vi "reg_visu.vi"(7 "name":string="GM10", 9 "stop":bool, 10 "connect (T)":bool=TRUE) -> (0 "error out":errorcluster, 5 "This VI":refnum<vi>)   [LabVIEW 2019]
uses:
  Heating/ctl/Z_ind_heating.ctl
  Heating/ctl/Z_Hswitch/Z_Hswitch.xctl
  ctl/Y/Y.xctl
  Heating/ctl/Z_State.ctl
  Heating/ctl/Y_state.ctl
  Heating/ctl/ZM_State.ctl
  Heating/ctl/Y_source.ctl
  ctl/control param simple.ctl
  ctl/Y_state.ctl
  ctl/Y_short.ctl
  Inputs/Ctl/Parameter State short.ctl
  ctl/ZY_control_short.ctl
  ctl/Z_State.ctl
  45230f51-ed9d-4592-a49a-e0edfe92ddd1.vi
  fbc51cc2-a17d-4d51-90ca-ef1d5e9adb43.vi
  81bac83f-5a8a-4521-9bb9-45d0222ee4c6.vi
  Y_switch_control.vi
  Y Limiter_ext.vi
  Counter/Generator simplified.vi
  <vilib>/NI/AMC/Create Single Message.vi
  <vilib>/NI/AMC/Update Message Routing Info.vi
  <vilib>/NI/AMC/Read Termination Message.vi
  PID Output Rate Limiter Ext.vi
  PID Timing Estimation Ext.vi
  Heating/Global stop.vi
  <vilib>/NI/AMC/Send Message.vi
  <vilib>/NI/AMC/Globals.vi
  Heating/Heating.lvlib
  <vilib>/NI/AMC/AMC.lvlib
  control.lvlib
  Inputs/Inputs.lvlib
panel:
  out "PV 2":dbl(slide) scale=0.0..1.0
  in  "Button":bool
  in  "Y":dbl step=0.01 format="%.2f"
  in  "Scale max":dbl=1.0 format="%#_13g"
  in  "name 4":string="Осн."
  in  "Unit":enum16{"l/h", "m3/h"}(ring)
  in  "name 3":string="Осн."
  in  "t":dbl=10.5 caption="сек."
  in  "alarm val":dbl=3.01 caption="m3/h"
  in  "auto":dbl=15.888 caption="Зависимый"
  in  "k":dbl=1.459 caption="Коэфф"
  in  "Y_SP":cluster{dbl, dbl, dbl}(xcontrol)
  in  "message name":string="AI redefine"
  out "status":string
  in  "process":bool
  in  "state variables":cluster{"CurrentFile":path}
  out "JSON string":string
  in  "JSON":string
  in  "Write controls":bool
  out "T stage":dbl format="%<%M:%S>t"
  in  "ALRL1_reset":bool
  in  "ALRL2_reset":bool
  out "Z3 ind":T1
  in  "Z_Hswitch":bool(xcontrol)
  out "Z5 State":string
  # "Время установки"
  # "Аварийный"
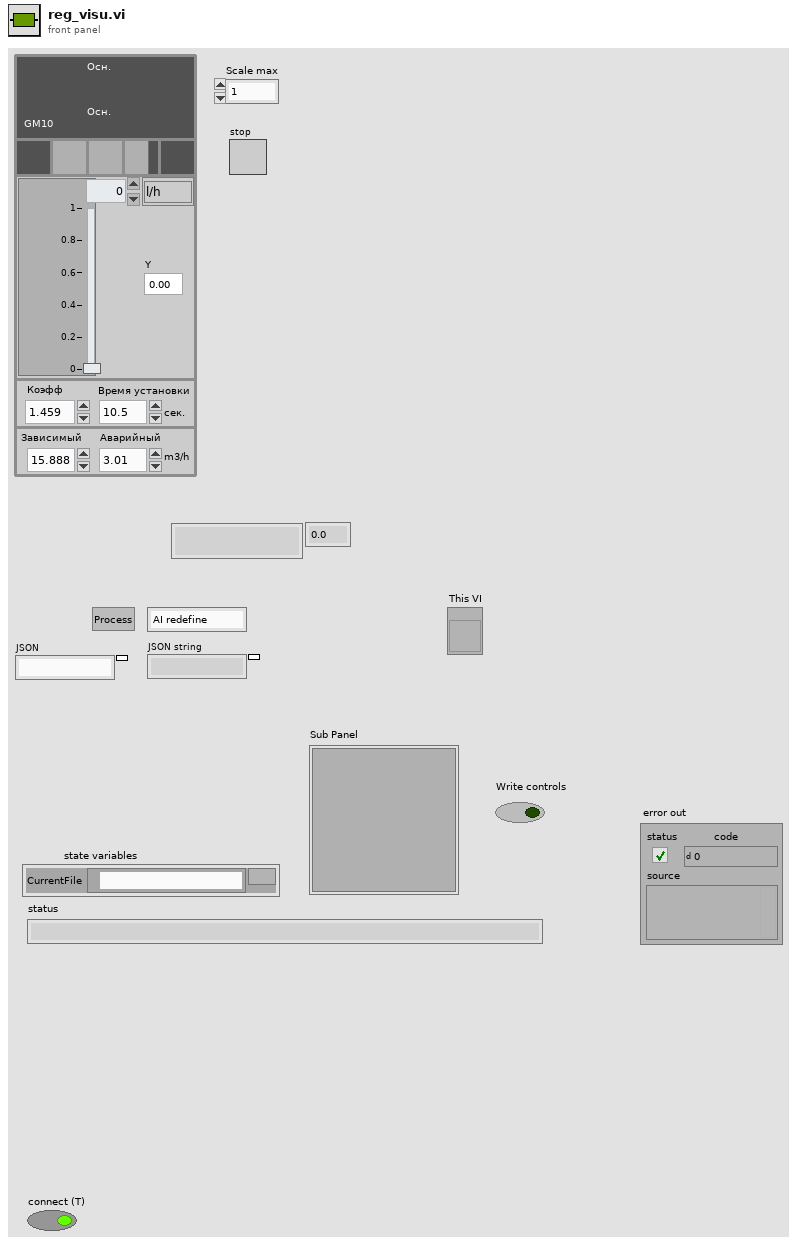
[diagram p1: front panel]
types:
  T1 = typedef "Heating.lvlib/Z_ind_heating.ctl" = u16
  T2 = typedef "AMC.lvlib/Message Queue.ctl" = refnum<queue>
  T3 = typedef "control.lvlib/ZY_control_short.ctl" = cluster{"Start":bool, "Z_HSw":u32, "Z_HSetState":T4, "Y_HSw":u32, "Y_HSetState":T5, "SP":dbl, "Y_H":dbl, "Y_A":dbl, "Reset_ALR":bool}
  T4 = typedef "control.lvlib/Z_State.ctl" = enum8{"initialization", "alarm", "disabled", "not ready", "stop ready", "reserv", "switched off", "reserv2", "switched on", "check", "on min", "decrease out", "on", "increase out", "on max"}
  T5 = typedef "control.lvlib/Y_state.ctl" = enum8{"initialize", "alarm", "min", "stop", "hand", "auto", "max"}
  T6 = typedef "control.lvlib/Y_short.ctl" = cluster{"Y_Source":u8, "Y_SetState":u8, "SP_Set":dbl, "SP":dbl, "PV":dbl, "PV_State":T7, "Y_preSet":dbl, "Y_Set":dbl, "Y":dbl, "Y_State":T7, "YB":bool}
  T7 = typedef "Inputs.lvlib/Parameter State short.ctl" = cluster{"code":i32, "visible":bool, "color":u32}
  T8 = cluster{"Y_HSw":u32, "Y_HSetState":T5, "Y_ASetState":T5, "Y_DSetState":T5}
  T9 = typedef "control.lvlib/control param simple.ctl" = cluster{"output high":dbl, "alr value":dbl, "output low":dbl, "output time (t)":dbl}
  T10 = typedef "Heating.lvlib/Y_source.ctl" = enum8{"initialize", "local disabled", "local hand", "hand", "auto", "dist"}
  T11 = cluster{"connect":bool, "SP_Source":T10, "SP_Set":dbl, "SP":dbl}
  T12 = typedef "Heating.lvlib/Y_state.ctl" = enum8{"initialize", "alarm", "min", "stop", "hand", "auto", "max"}
  T13 = typedef "Heating.lvlib/Z_State.ctl" = enum8{"initialization", "alarm", "disabled", "not ready", "stop ready", "reserv", "switched off", "reserv2", "switched on", "check", "on min", "decrease out", "on", "increase out", "on max"}
  T14 = typedef "Heating.lvlib/ZM_State.ctl" = enum8{"initialization", "stop", "start_cmd", "contactor_on_cmd", "heating", "on", "stop_cmd", "power_down", "contactor_off_cmd", "cooling", "restart_delay"}
  T15 = enum32{"Invalid Status", "Unconnected", "Active", "Idle", "Error", "Connecting"}
  T16 = typedef "LVDataSocketStatusTypeDef.ctl" = cluster{"Code":enum32{"Invalid Status", "Unconnected", "Active", "Idle", "Error", "Connecting"}, "Text":string}
  T17 = typedef "Y_Lim_ext_defs.ctl" = cluster{"reinitialize":bool, "SpLim_State":T18, "output":dbl, "Tick":u32, "output rate":dbl, "Y_Set":dbl, "Y_preSet":dbl}
  T18 = typedef "Y_Lim_State.ctl" = enum8{"initialization", "alarm", "stop", "decrease", "increase"}
  T19 = typedef "control.lvlib/Y.ctl" = cluster{"Y_Source":T20, "Y_SetState":T5, "SP_Set":dbl, "SP":dbl, "PV":dbl, "PV_State":T7, "Y_preSet":dbl, "Y_Set":dbl, "Y":dbl, "Y_State":T7, "YB":bool}
  T20 = typedef "control.lvlib/Y_source.ctl" = enum8{"initialize", "local disabled", "local hand", "hand", "auto", "dist"}
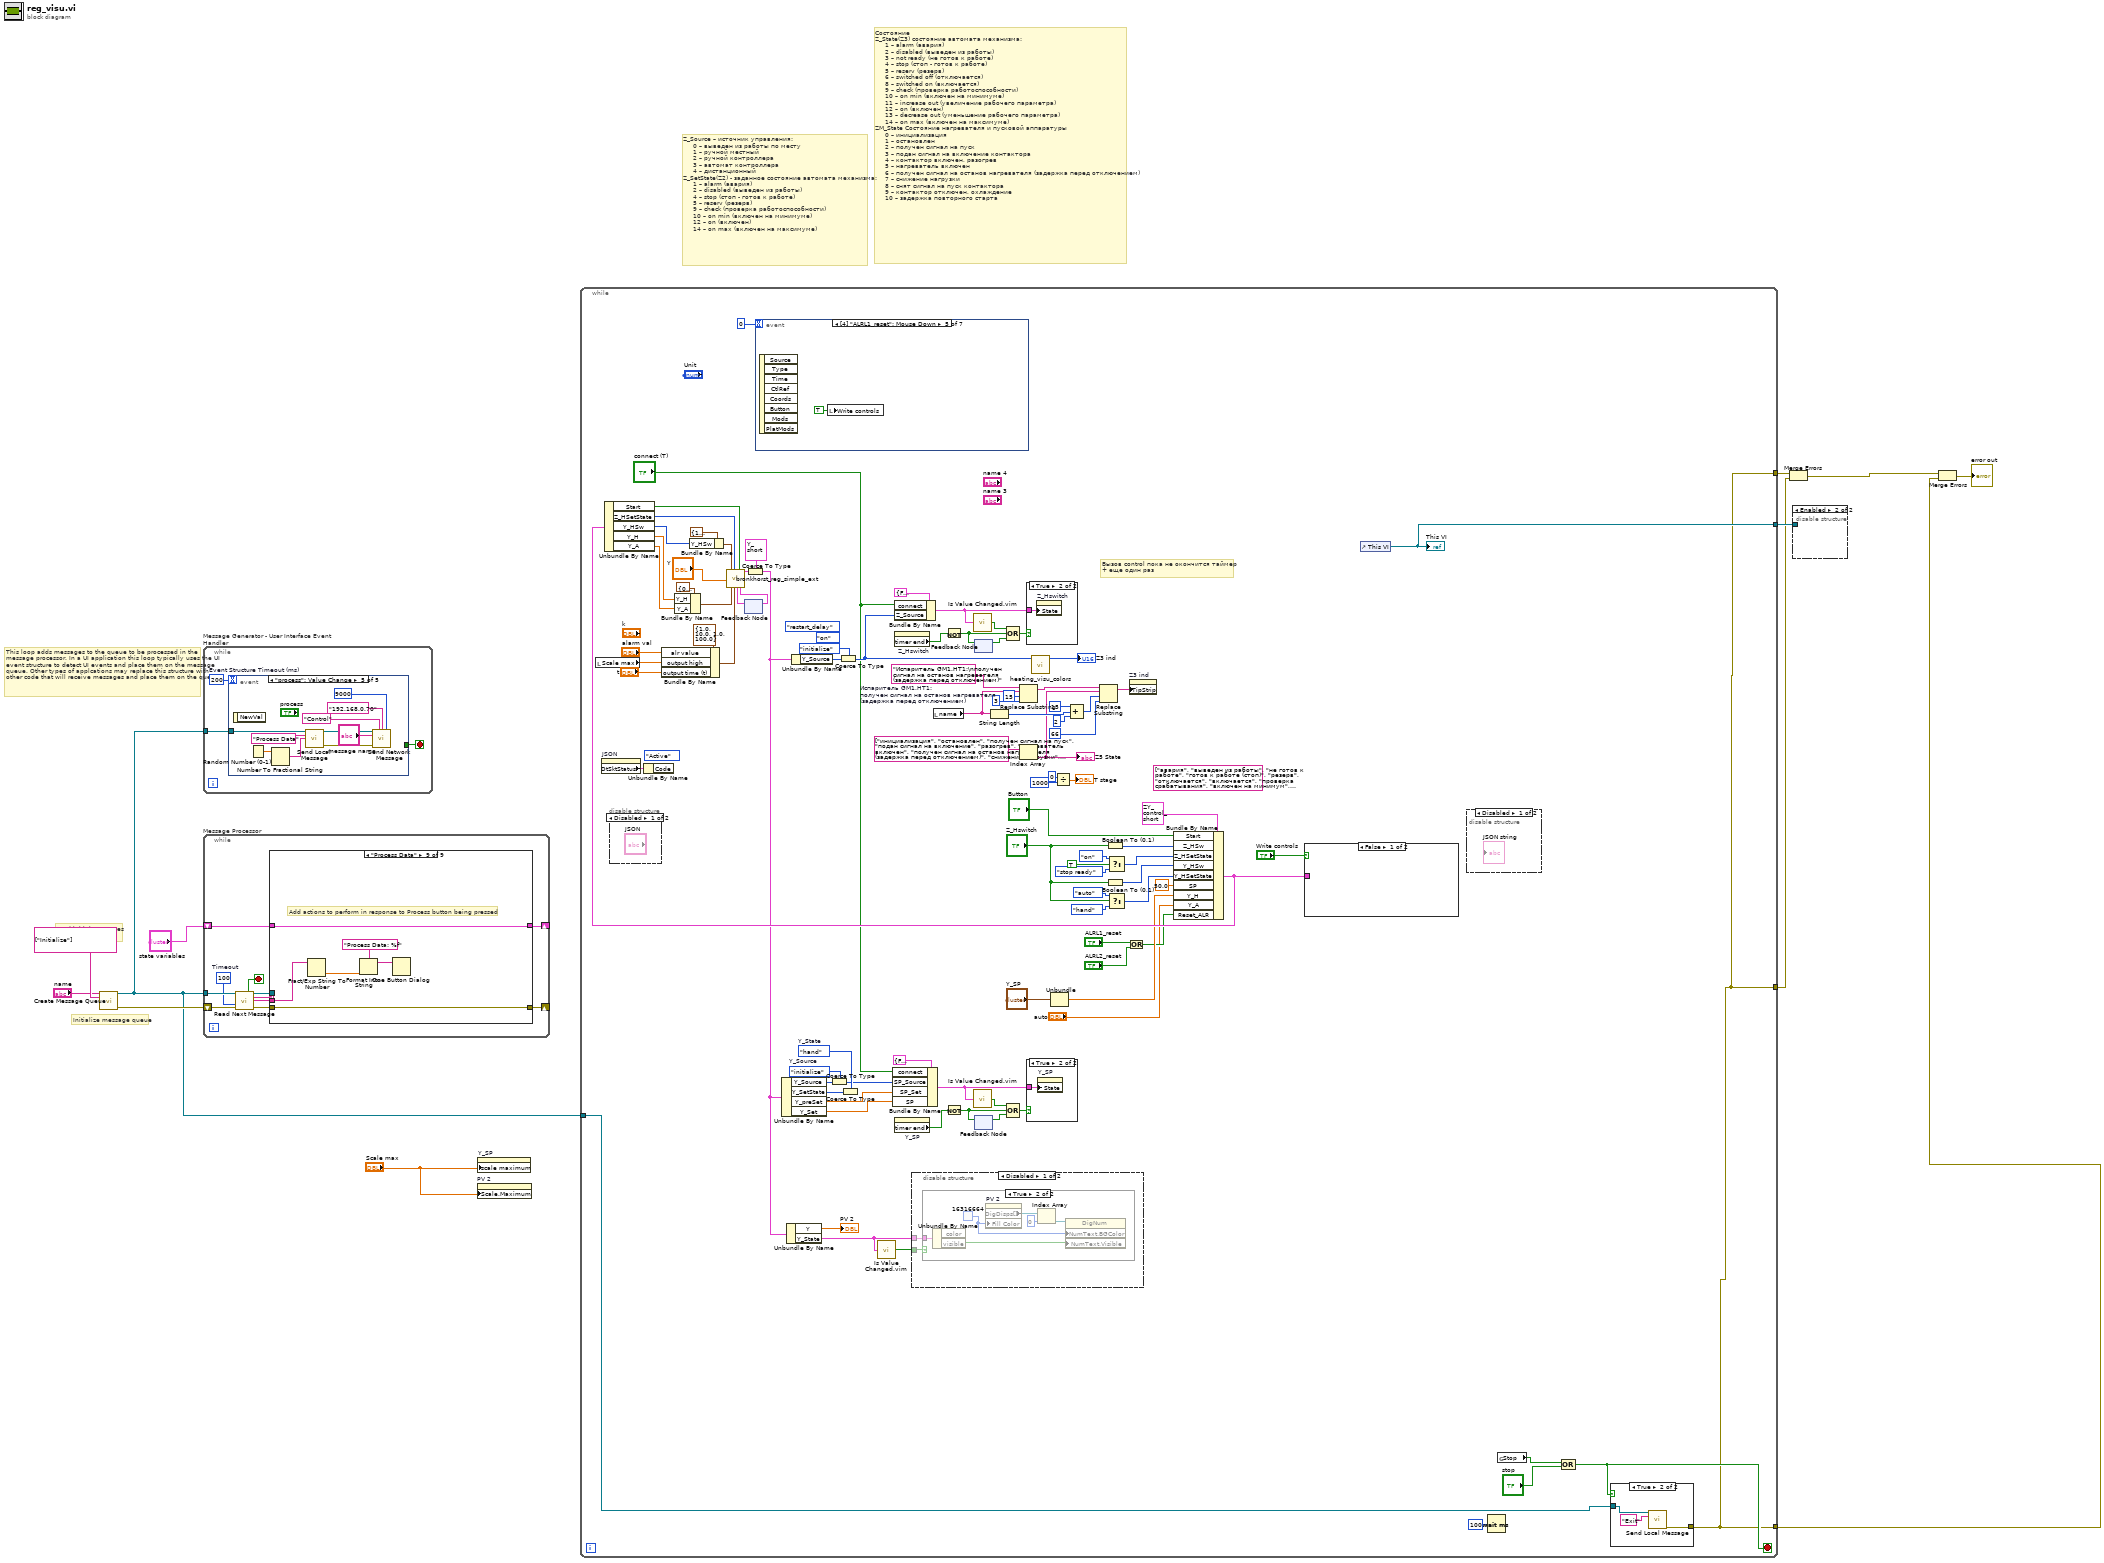
[diagram p0: block diagram]
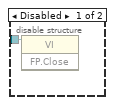
[diagram p2: hidden frame]
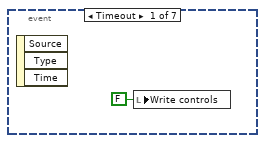
[diagram p8: hidden frame]
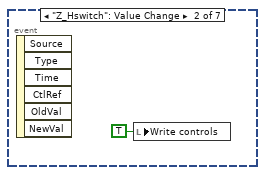
[diagram p9: hidden frame]
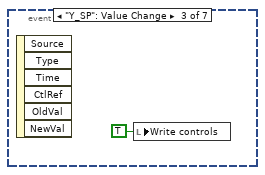
[diagram p10: hidden frame]
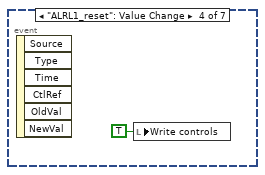
[diagram p11: hidden frame]
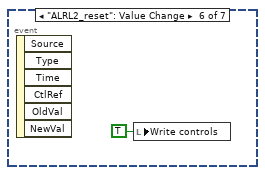
[diagram p12: hidden frame]
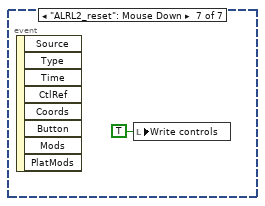
[diagram p13: hidden frame]
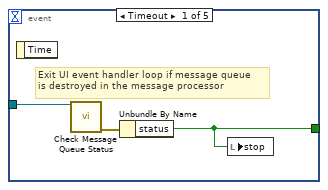
[diagram p17: hidden frame]
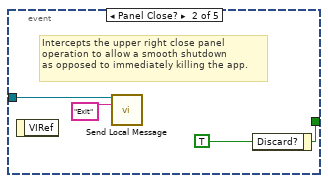
[diagram p18: hidden frame]
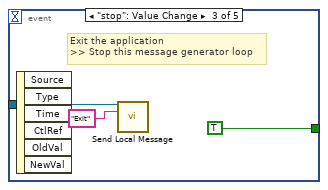
[diagram p19: hidden frame]
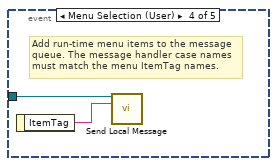
[diagram p20: hidden frame]
diagram:
  # "This loop adds messages to the queue to be processed in the message processor. In a UI application this loop typically uses the UI event structure to detect UI events and place them on the message queue. Other types of applcations may replace this structure with other code that will receive messages and place them on the queue."
  # "Initialize message queue"
  # "Load initial messages\non the queue"
  # "Состояние\nZ_State(Z3) состояние автомата механизма:\n     1 – alarm (авария)\n     2 – disabled (выведен из работы)\n     3 – not ready (не готов к работе)\n     4 – stop (стоп - готов к работе)\n     5 – reserv (резерв)\n     6 – switched off (отключается)\n     8 – switched on (включается)\n     9 – check (проверка работоспособности)\n     10 – on min (включен на минимуме)\n     11 – increase out (увеличение рабочего параметра)\n     12 – on (включен)\n     13 – decrease out (уменьшение рабочего параметра)\n     14 – on max (включен на максимуме)\nZM_State Состояние нагревателя и пусковой аппаратуры\n     0 – инициализация\n     1 – остановлен\n     2 – получен сигнал на пуск\n     3 – подан сигнал на включение контактора\n     4 – контактор включен, разогрев\n     5 – нагреватель включен\n     6 – получен сигнал на останов нагревателя (задержка перед отключением)\n     7 – снижение нагрузки\n     8 – снят сигнал на пуск контактора\n     9 – контактор отключен, охлаждение\n     10 – задержка повторного старта"
  # "Z_Source – источник управления:\n     0 – выведен из работы по месту\n     1 – ручной местный\n     2 – ручной контроллера\n     3 – автомат контроллера\n     4 – дистанционный\nZ_SetState(Z2) - заданное состояние автомата механизма:\n     1 – alarm (авария)\n     2 – disabled (выведен из работы)\n     4 – stop (стоп - готов к работе)\n     5 – reserv (резерв)\n     9 – check (проверка работоспособности)\n     10 – on min (включен на минимуме)\n     12 – on (включен)\n     14 – on max (включен на максимуме)"
  n1 = call <vilib>:"Create Message Queue.vi"("message queue name"="name", "initial message names"=string[] ["Initialize"]) -> ("message queue out"=w6:T2, "error out"=w8:errorcluster)  [unwired: 12 in]
  n2 = while "Message Generator - User Interface Event Handler" {
    tunnel: w6 -> [w13]
    stop <- w14 stop-if-true
    w15 = 200  # Event Structure Timeout (ms)
    n3 = event shown="[4] \"process\": Value Change" {
      selector: _ -> [_ _ _ _ _]
      dyn-events: _ -> [_ _ _ _ _]
      timeout: w15 -> [_ _ _ _ _]
      tunnel: [w16 w21 TRUE ("Discard?") _ _] -> w14
      tunnel: w13 -> [w17 w19 w22 w25 w36]
      event Timeout {
        # "Exit UI event handler loop if message queue\nis destroyed in the message processor"
        n4 = event-data() -> ()  [unwired: 2 out]
        n5 = call <vilib>:"Check Message Queue Status.vi"("message queue in"=w17) -> ("error out"=w18:errorcluster)  [unwired: 10 in, 4 out]
        n6 = Unbundle By Name(w18) -> ("status"=w16:bool)
        n7 = local write "stop"(w16) -> ()
      }
      event Panel Close? {
        w21 = TRUE ("Discard?")
        # "Intercepts the upper right close panel\noperation to allow a smooth shutdown\nas opposed to immediately killing the app."
        n8 = event-data() -> ()  [unwired: 2 out]
        n9 = call <vilib>:"Send Local Message.vi"("message queue in"=w19, "message name"="Exit") -> ()  [unwired: 11 in, 3 out]
        n10 = event-data("Discard?"=w21) -> ()  [unwired: 1 in, 1 out]
      }
      event "stop": Value Change {
        # "Exit the application\n>> Stop this message generator loop"
        n11 = event-data() -> ()  [unwired: 7 out]
        n12 = call <vilib>:"Send Local Message.vi"("message queue in"=w22, "message name"="Exit") -> ()  [unwired: 11 in, 3 out]
      }
      event Menu Selection (User) {
        # "Add run-time menu items to the message\nqueue. The message handler case names must match the menu ItemTag names."
        n13 = event-data() -> ("ItemTag"=w26:string)  [unwired: 1 out]
        n14 = call <vilib>:"Send Local Message.vi"("message queue in"=w25, "message name"=w26) -> ()  [unwired: 11 in, 3 out]
      }
      event "process": Value Change {
        n15 = event-data() -> ()  [unwired: 2 out]
        n16 = Random Number (0-1)() -> (number: 0 to 1=w33:dbl)
        n17 = Number To Fractional String(number=w33) -> (F-format string=w34:string)  [unwired: 3 out]
        n18 = call <vilib>:"Send Local Message.vi"("message queue in"=w36, "message name"="Process Data", "message value"=w34) -> ("message queue out"=w32:T2, "error out"=w28:errorcluster)  [unwired: 10 in, 1 out]
        n19 = call <vilib>:"Send Network Message.vi"("message queue in"=w32, "receiver process"="Control", "receiver host"="192.168.0.70", "receiver port (0)"=u16 9000, "message name"="message name", "error in"=w28) -> ()  [unwired: 7 in, 3 out]
      }
    }
  }
  n20 = while "Message Processor" {
    shift-left: w8 -> [w41]
    shift-right: [w45] -> _
    tunnel: w6 -> [w42]
    shift-left: "state variables" -> [w47]
    shift-right: [w46] -> _
    stop <- w44 stop-if-true
    w37 = 100  # Timeout
    n21 = call <vilib>:"Read Next Message.vi"("message queue in"=w42, "timeout (1 ms)"=w37, "error in"=w41) -> ("exit process?"=w44:bool, "message queue out"=w43:T2, "message name"=w39:string, "message value"=w38:string, "error out"=w40:errorcluster)  [unwired: 5 in, 3 out]
    n22 = case shown="\"Process Data\"" w39 {
      selector: w39 -> [_ _ w59 _ _ _ _ _ _]
      tunnel: [w49 w56 w61 w66 w68 w70 w75 w77 w82] -> w46
      tunnel: w47 -> [w49 w56 w61 w66 w68 w70 w75 w77 w82]
      tunnel: w43 -> [_ _ _ w64 _ _ w72 _ _]
      tunnel: w40 -> [w48 w55 w60 w62 w67 w69 w73 w76 w83]
      tunnel: [w48 w55 w60 errorcluster {"status"=FALSE, "code"=0, "source"=""} ("error out") w67 w69 w71 w76 w83] -> w45
      tunnel: w38 -> [_ _ _ _ _ _ _ _ w81]
      frame "---------- Framework Operations ----------" {
        # "Dummy case to add a seperator in the Case Structure menu"
      }
      frame "", "Idle" {
        # "Update the front panel"
        # "Idle Case - this case is called after a Timeout on the Get Next Message from Queue VI, if no new messages are present on the queue. This case can be used for housekeeping tasks such as updating the UI."
        n23 = Get Date/Time String(want seconds? (F)=TRUE) -> (date string=w54:string, time string=w53:string)  [unwired: 2 out]
        n24 = Concatenate Strings(w54, " " ("string"), w53) -> (→"status":string)
      }
      frame "Missing Message Handler", Default {
        # "Call this case if a message is received that is not handled \nby any other case. Typically this is a programming error\nas a result of a typo or unhandled message/missing message handler."
        n25 = Format Into String(format string="DevError: Missing message handler for '%s\" message." ("message"), w59) -> (resulting string=w57:string)  [unwired: 2 in, 1 out]
        n26 = One Button Dialog(message=w57) -> ()  [unwired: 2 out]
      }
      frame "Error" {
        # "Proceed to Exit - Remove this if it is\nnot appropriate for the General Error case"
        # "General Error Case - this case is called if an error is passed using the error cluster below. Typically most new errors should be handed in each individual case and not passed in the rror cluster. If necessary a custom error handler case should be added and called from other cases."
        n27 = call <vilib>:"Simple Error Handler.vi"("error in (no error)"=w62) -> ()  [unwired: 1 in, 8 out]
        n28 = call <vilib>:"Send Local Message.vi"("message queue in"=w64, "message name"="Exit") -> ()  [unwired: 11 in, 3 out]
      }
      frame "---------- Generic Operations ----------" {
        # "Dummy case to add a seperator in the Case Structure menu"
      }
      frame "Initialize" {
        # "Initialize the state variables and user interface"
      }
      frame "Exit" {
        # "Destroy message queue >> this will halt the UI event handler loop"
        # "Stop the VI\n>> Perform any cleanup tasks in this message case.\n>> Clear display before closing."
        n29 = call <vilib>:"Destroy Message Queue.vi"("message queue in"=w72, "error in"=w73) -> ("error out"=w71:errorcluster)  [unwired: 11 in, 2 out]
        n30 = local write "status"("" ("Status")) -> ()
      }
      frame "---------- Application Operations ----------" {
        # "Dummy case to add a seperator in the Case Structure menu"
      }
      frame "Process Data" {
        # "Add actions to perform in response to Process button being pressed"
        n31 = Fract/Exp String To Number(string=w81) -> (number=w80:dbl)  [unwired: 4 out]
        n32 = Format Into String(format string="Process Data: %f" ("message"), w80) -> (resulting string=w78:string)  [unwired: 2 in, 1 out]
        n33 = One Button Dialog(message=w78) -> ()  [unwired: 2 out]
      }
    }
  }
  n34 = property on="PV 2" class="Slide (strict)"("Scale.Maximum"="Scale max") -> ()  [unwired: 2 in, 2 out]
  n35 = property on="Y_SP" class="Y (strict)"("scale maximum"="Scale max") -> ()  [unwired: 2 in, 2 out]
  n36 = while {
    tunnel: [w147] -> w12
    tunnel: [w114] -> w11
    tunnel: [w114] -> w10
    tunnel: w6 -> [w145]
    tunnel: [w114] -> w5
    stop <- w146 stop-if-true
    w138 = Y_state."hand"  # Y_State
    w139 = Y_source."initialize"  # Y_Source
    (unwired) ZM_State."restart_delay" ("ZM_State_heating")
    (unwired) Z_State."on" ("Z_State_heating")
    (unwired) T15."Active" ("Code")
    (unwired) string[] ["авария", "выведен из работы", "не готов к работе", "готов к работе (стоп)", "резерв", "отключается", "включается", "проверка срабатывания", "включен на минимум", "увеличение произв", "включен", "уменьшение произв", "включен на максимум"]
    w175 = "Испаритель GM1.HT1:\nполучен сигнал на останов нагревателя (задержка перед отключением)"  # Испаритель GM1.HT1: получен сигнал на останов нагревателя (задержка перед отключением)
    # "Вызов control пока не окончится таймер\n+ еще один раз"
    n37 = local read "Scale max"() -> (w106:dbl)
    n38 = property on="JSON" class="Str"() -> ("DtSktStatus"=w148:T16)  [unwired: 2 in, 2 out]
    n39 = disable-structure shown="Disabled" {
      frame Disabled {
      }
      frame Enabled {
      }
    }
    n40 = Unbundle By Name(w148) -> ()  [unwired: 1 out]
    n41 = Bundle By Name(cluster=T9 {"output high"=1.0, "alr value"=10.0, "output low"=1.0, "output time (t)"=100.0} ("control param"), "alr value"="alarm val", "output high"=w106, "output time (t)"="t") -> (w104:T9)
    n42 = feedback #1() -> (w91:T17)  [unwired: 1 in]
    n43 = event shown="[4] \"ALRL1_reset\": Mouse Down" {
      selector: _ -> [_ _ _ _ _ _ _]
      dyn-events: _ -> [_ _ _ _ _ _ _]
      timeout: 0 -> [_ _ _ _ _ _ _]
      event Timeout {
        n44 = event-data() -> ()  [unwired: 1 in, 3 out]
        n45 = local write "Write controls"(FALSE ("manual_reset")) -> ()
      }
      event "Z_Hswitch": Value Change {
        n46 = event-data() -> ()  [unwired: 1 in, 6 out]
        n47 = local write "Write controls"(TRUE ("manual_reset")) -> ()
      }
      event "Y_SP": Value Change {
        n48 = event-data() -> ()  [unwired: 1 in, 6 out]
        n49 = local write "Write controls"(TRUE ("manual_reset")) -> ()
      }
      event "ALRL1_reset": Value Change {
        n50 = event-data() -> ()  [unwired: 1 in, 6 out]
        n51 = local write "Write controls"(TRUE ("manual_reset")) -> ()
      }
      event "ALRL1_reset": Mouse Down {
        n52 = event-data() -> ()  [unwired: 1 in, 8 out]
        n53 = local write "Write controls"(TRUE ("manual_reset")) -> ()
      }
      event "ALRL2_reset": Value Change {
        n54 = event-data() -> ()  [unwired: 1 in, 6 out]
        n55 = local write "Write controls"(TRUE ("manual_reset")) -> ()
      }
      event "ALRL2_reset": Mouse Down {
        n56 = event-data() -> ()  [unwired: 1 in, 8 out]
        n57 = local write "Write controls"(TRUE ("manual_reset")) -> ()
      }
    }
    n58 = property on="Z_Hswitch" class="Z_Hswitch (strict)"() -> ("timer end"=w129:bool)  [unwired: 2 in, 2 out]
    n59 = property on="Y_SP" class="Y (strict)"() -> ("timer end"=w126:bool)  [unwired: 2 in, 2 out]
    n60 = local read "name"() -> (w144:string)
    n61 = Not(x=w129) -> (.not. x?=w133:bool)
    n62 = Not(x=w126) -> (.not. x?=w124:bool)
    n63 = feedback #2() -> (w132:bool)  [unwired: 1 in]
    n64 = feedback-in #2(w133) -> ()
    n65 = feedback #3() -> (w123:bool)  [unwired: 1 in]
    n66 = feedback-in #3(w124) -> ()
    n67 = String Length(string=w144) -> (length=w170:i32)
    n68 = Index Array(array=string[] ["инициализация", "остановлен", "получен сигнал на пуск", "подан сигнал на включение", "разогрев", "нагреватель включен", "получен сигнал на останов нагревателя (задержка перед отключением)", "снижение нагрузки", "снят сигнал на пуск", "охлаждение", "задержка повторного старта"]) -> (element=w163:string)  [unwired: 1 in]
    "Z5 State" <- w163
    n69 = Replace Substring(2:3 ("length (len. of substring)"), 3:15 ("offset (0)"), 4:w144, 5:w175) -> (1:w172:string)  [unwired: 1 out]
    n70 = Unbundle("Y_SP") -> (w97:dbl)  [unwired: 2 out]
    n71 = Divide(x=u32 0, y=u32 1000) -> (x/y=→"T stage":dbl)
    n72 = Compound Arithmetic op=ADD(15 ("offset (0)"), w170, 2 ("value")) -> (w168:i32)
    n73 = Replace Substring(2:66 ("value"), 3:w168, 4:w163, 5:w172) -> (1:w167:string)  [unwired: 1 out]
    n74 = Boolean To (0,1)(Boolean="Z_Hswitch") -> (0, 1=w159:i16)
    n75 = Boolean To (0,1)(Boolean="Z_Hswitch") -> (0, 1=w156:i16)
    n76 = Select(t=Z_State."on" ("Z_State"), s=TRUE, f=Z_State."stop ready" ("Z_State")) -> (s? t:f=w162:T13)
    n77 = Select(t=Y_state."auto" ("Y_HSetState"), s="Z_Hswitch", f=Y_state."hand" ("Y_HSetState")) -> (s? t:f=w153:T12)
    n78 = Or(x="ALRL1_reset", y="ALRL2_reset") -> (x .or. y?=w86:bool)
    n79 = property on="Z3 ind" class="Ring (strict)"("TipStrip"=w167) -> ()  [unwired: 2 in, 2 out]
    n80 = Bundle By Name(cluster=T3 {"Start"=FALSE, "Z_HSw"=1, "Z_HSetState"=enum."on", "Y_HSw"=1, "Y_HSetState"=enum."hand", "SP"=0.0, "Y_H"=0.0, "Y_A"=0.0, "Reset_ALR"=FALSE} ("ZY_control"), "Start"="Button", "Z_HSw"=w159, "Z_HSetState"=w162, "Y_HSw"=w156, "Y_HSetState"=w153, "SP"=50.0, "Y_H"=w97, "Y_A"="auto", "Reset_ALR"=w86) -> (w113:T3)
    n81 = Unbundle By Name(w113) -> ("Start"=w87:bool, "Z_HSetState"=w90:T4, "Y_HSw"=w101:u32, "Y_H"=w110:dbl, "Y_A"=w84:dbl)
    n82 = Bundle By Name(cluster=cluster{"Y_H":dbl, "Y_A":dbl, "Y_D":dbl} {"Y_H"=0.0, "Y_A"=0.0, "Y_D"=0.0} ("controls Y"), "Y_H"=w110, "Y_A"=w84) -> (w109:cluster{"Y_H":dbl, "Y_A":dbl, "Y_D":dbl})
    n83 = Bundle By Name(cluster=T8 {"Y_HSw"=1, "Y_HSetState"=enum."hand", "Y_ASetState"=enum."hand", "Y_DSetState"=enum."auto"} ("Y_Set"), "Y_HSw"=w101) -> (w100:T8)
    n84 = call "bronkhorst_reg_simple_ext.vi"("Y"="Y", "Y_Set"=w100, "controls Y"=w109, "Z"=w90, "control param"=w104, "Y_limiter_old"=w91, "Start"=w87) -> ("Y_limiter"=w92:T17, "Y_State"=w94:T19)  [unwired: 8 in, 3 out]
    n85 = feedback-in #1(w92) -> ()
    n86 = Coerce To Type(0:w94, 1:T6 {"Y_Source"=1, "Y_SetState"=5, "SP_Set"=0.0, "SP"=0.0, "PV"=0.0, "PV_State"={"code"=0, "visible"=FALSE, "color"=0}, "Y_preSet"=0.0, "Y_Set"=0.0, "Y"=0.0, "Y_State"={"code"=0, "visible"=FALSE, "color"=0}, "YB"=FALSE} ("Y_State")) -> (2:w93:T6)
    n87 = Unbundle By Name(w93) -> ("Y_Source"=w141:u8, "Y_SetState"=w157:u8, "Y_preSet"=w99:dbl, "Y_Set"=w98:dbl)
    n88 = Unbundle By Name(w93) -> ("Y"=→"PV 2":dbl, "Y_State"=w128:T7)
    n89 = Unbundle By Name(w93) -> ("Y_Source"=w142:u8)
    n90 = Coerce To Type(0:w141, 1:w139) -> (2:w117:T10)
    n91 = Coerce To Type(0:w142, 1:Y_source."initialize" ("Y_Source")) -> (2:w137:T10)
    n92 = Coerce To Type(0:w157, 1:w138) -> ()  [unwired: 1 out]
    n93 = call "Is Value Changed.vim"("value"=w128) -> ("changed or first call?"=w135:bool)
    n94 = Bundle By Name(cluster=T11 {"connect"=FALSE, "SP_Source"=enum."initialize", "SP_Set"=0.0, "SP"=0.0} ("source"), "connect"="connect (T)", "SP_Source"=w117, "SP_Set"=w99, "SP"=w98) -> (w127:T11)
    n95 = Bundle By Name(cluster=cluster{"connect":bool, "Z_Source":T10} {"connect"=FALSE, "Z_Source"=enum."initialize"} ("source"), "connect"="connect (T)", "Z_Source"=w137) -> (w130:cluster{"connect":bool, "Z_Source":T10})
    n96 = disable-structure shown="Disabled" {
      disable-tunnel: w135 -> [w180 _]
      disable-tunnel: w128 -> [w179 _]
      frame Disabled {
        n97 = case shown="True" w180 {
          tunnel: w179 -> [_ w182]
          frame False {
          }
          frame True {
            w181 = u32 16316664 ("Color Box")
            n98 = Unbundle By Name(w182) -> ("visible"=w183:bool)  [unwired: 1 out]
            n99 = property on="PV 2" class="Slide (strict)"("Fill Color"=w181) -> ("DigDisps[]"=w186:refnum<vi>[])  [unwired: 2 in, 2 out]
            n100 = Index Array(array=w186, index=0) -> (element=w184:refnum<vi>)
            n101 = property on="Property Node" class="DigNum"(reference=w184, "NumText.BGColor"=w181, "NumText.Visible"=w183) -> ()  [unwired: 1 in, 2 out]
          }
        }
      }
      frame Enabled {
      }
    }
    n102 = call "Is Value Changed.vim"("value"=w130) -> ("changed or first call?"=w134:bool)
    n103 = call "Is Value Changed.vim"("value"=w127) -> ("changed or first call?"=w125:bool)
    n104 = Compound Arithmetic op=OR(w134, w133, w132) -> (w131:bool)
    n105 = Compound Arithmetic op=OR(w125, w124, w123) -> (w122:bool)
    n106 = case shown="True" w131 {
      tunnel: w130 -> [_ w188]
      frame False {
      }
      frame True {
        n107 = property on="Z_Hswitch" class="Z_Hswitch (strict)"("State"=w188) -> ()  [unwired: 2 in, 2 out]
      }
    }
    n108 = case shown="True" w122 {
      tunnel: w127 -> [_ w187]
      frame False {
      }
      frame True {
        n109 = property on="Y_SP" class="Y (strict)"("State"=w187) -> ()  [unwired: 2 in, 2 out]
      }
    }
    n110 = call "heating_visu_colors.vi"("Z_Source"=w137) -> ("N ring"=→"Z3 ind":u16)  [unwired: 7 in, 3 out]
    n111 = case shown="False" "Write controls" {
      tunnel: w113 -> [_ _]
      frame False {
      }
      frame True {
      }
    }
    n112 = control-ref of="This VI"() -> (w147:refnum<vi>)
    "This VI" <- w147
    n113 = disable-structure shown="Disabled" {
      frame Disabled {
      }
      frame Enabled {
      }
    }
    n114 = Wait (ms)(milliseconds to wait=u32 100) -> ()  [unwired: 1 out]
    n115 = global read "Global stop.vi" "Stop"() -> (w150:bool)
    n116 = Compound Arithmetic op=OR(w150, "stop") -> (w146:bool)
    n117 = case shown="True" w146 {
      tunnel: w145 -> [_ w197]
      tunnel: [_ w196] -> w114
      frame False {
      }
      frame True {
        n118 = call <vilib>:"Send Local Message.vi"("message queue in"=w197, "message name"="Exit") -> ("error out"=w196:errorcluster)  [unwired: 11 in, 2 out]
      }
    }
  }
  n119 = Merge Errors(w10, w11) -> (w1:errorcluster)
  n120 = disable-structure shown="Enabled" {
    disable-tunnel: w12 -> [w199 _]
    frame Disabled {
      n121 = invoke class="VI" method="FP.Close"(reference=w199) -> ()  [unwired: 2 in, 3 out]
    }
    frame Enabled {
    }
  }
  n122 = Merge Errors(w1, w5) -> (→"error out":errorcluster)
